vi "exercise 1-2.vi"() -> ()   [LabVIEW 2018]
panel:
  in  "문자열":string
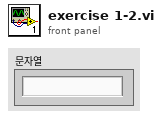
[diagram p1: front panel]
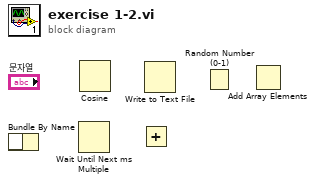
[diagram p0: block diagram]
diagram:
  n1 = Bundle By Name() -> ()  [unwired: 2 in, 1 out]
  n2 = Wait Until Next ms Multiple() -> ()  [unwired: 1 in, 1 out]
  n3 = Cosine() -> ()  [unwired: 1 in, 1 out]
  n4 = Add() -> ()  [unwired: 2 in, 1 out]
  n5 = Write to Text File() -> ()  [unwired: 4 in, 3 out]
  n6 = Random Number (0-1)() -> ()  [unwired: 1 out]
  n7 = Add Array Elements() -> ()  [unwired: 1 in, 1 out]
